vi "test_fpga_ort_fit.vi"() -> ()   [LabVIEW 2016]
uses:
  <vilib>/Platform/TimedLoop/XDataNode/timing_clust.ctl
  <vilib>/Platform/TimedLoop/XDataNode/nitl_modes.ctl
  <vilib>/Platform/TimedLoop/XDataNode/wakeup.ctl
  <vilib>/rvi/Emulation/niFpgaSctlEmulationGetInTimedLoop.vi
  <vilib>/rvi/Emulation/niFpgaEmulationReportErrorSimple.vi
  <vilib>/rvi/Emulation/niFpgaGetClockAttributes.vi
  <vilib>/rvi/Emulation/niFpgaCriticalErrorInLSC.vi
  <vilib>/rvi/Emulation/niFpgaProcessEmulError.vi
  <vilib>/rvi/Emulation/niFpgaEmulationIsFPGAContextNoSignature.vi
  <vilib>/rvi/DataTransferAndStorage/Container/Common/niFpgaContainerGetUniqueNameForEmu.vi
  <vilib>/rvi/Memory/Memory_Emulation/niFpgaMemoryEmulationCacheClearOnFirstRun.vi
  <vilib>/rvi/Memory/Memory_Emulation/nirvimemoryEmulationManagerCache_MakeExclusive.vi
  <vilib>/rvi/Memory/Memory_Emulation/niFpgaMemoryEmulationValidateCache.vi
  <vilib>/rvi/Memory/Memory_Emulation/nirvimemoryEmulationManagerCache_InsertValue.vi
  <vilib>/Utility/error.llb/Clear Errors.vi
  <vilib>/rvi/Memory/Memory_Emulation/nirvimemoryEmulationManagerCache_ReleaseExclusive.vi
  <vilib>/rvi/Memory/Memory_Emulation/nirvimemoryEmulationManagerCache_GetValue.vi
  <vilib>/rvi/Memory/Memory_Emulation/nirvimemoryEmulationManagerCache_SetValue.vi
  <vilib>/rvi/Memory/Memory_Emulation/nirvimemoryFastEmulation.vi
  <vilib>/rvi/Memory/Memory_Emulation/nirvimemoryEmulation.vi
  <vilib>/rvi/errors/nirviReportUnexpectedCaseInternalError (U32).vi
  <vilib>/Platform/TimedLoop/XDataNode/XDataNode.xnode
  <vilib>/rvi/DataTransferAndStorage/Container/XNode/niFpgaContainer.xnode
  <vilib>/rvi/DataTransferAndStorage/Register/Emulation/niFpgaRegisterEmulation.vi
  <vilib>/Platform/TimedLoop/XDataNode/XDNodeRunTimeDep.lvlib
  <vilib>/rvi/FIFO/Fifo_Resource/nirvififoEmulationRead.vi
  <vilib>/rvi/DataTransferAndStorage/Handshake/Emulation/niFpgaHandshakeEmulation.vi
  <vilib>/rvi/FIFO/Fifo_Resource/nirvififoEmulationWrite.vi
panel:
  out "expMABundle":T1
  out "debugOutFitIntermediate":T2
  in  "ort.fit.m.coefficients":T3
  in  "ort.fit.m.weights":T4
  out "paramExtractDebug":cluster{"index":u16, "minimum":i16}
  in  "auxIn":i16
  in  "auxInValid":bool
  in  "inElementValid":bool=TRUE
  in  "inElement":cluster{"index":u16, "data":i16}
  out "debugOutSlopeDissi":T5
  in  "endOfCycle":bool=TRUE
  out "procVar":T6
  in  "ort.fit.p.params":T7={"maxLoc"=0, "threshold"=0, "fitHardPtLimit"=5000}
  in  "ort.p.waveSize":u16=5000
  in  "ort.bgc.p.bgCntP2":u16=12
  out "ort.o.maxIndex":u16
  out "aio.s.ortSubstDeflection":cluster{"index":u16, "data":i16}
  out "ort.o.interactionMax":fxp<+/-,24,16>
  in  "ort.p.fcAvgEnable":bool
  in  "ort.p.fcAvg":i8=-4
  in  "ort.p.methodParams":T8={"ort.p.winSizeP2"=2, "ort.p.syncPoint"=0, "ort.p.useSyncPoint"=FALSE, "ort.p.bypassAvg"=FALSE, "ort.p.searchBounds"={"maxSearchLower"=200, "maxSearchUpper"=600}}
  in  "fb.i.source":u8(ring) items=["Contact Mode", "ORT", "Aux"]
  in  "aio.i.samplingDecimation":u16=1
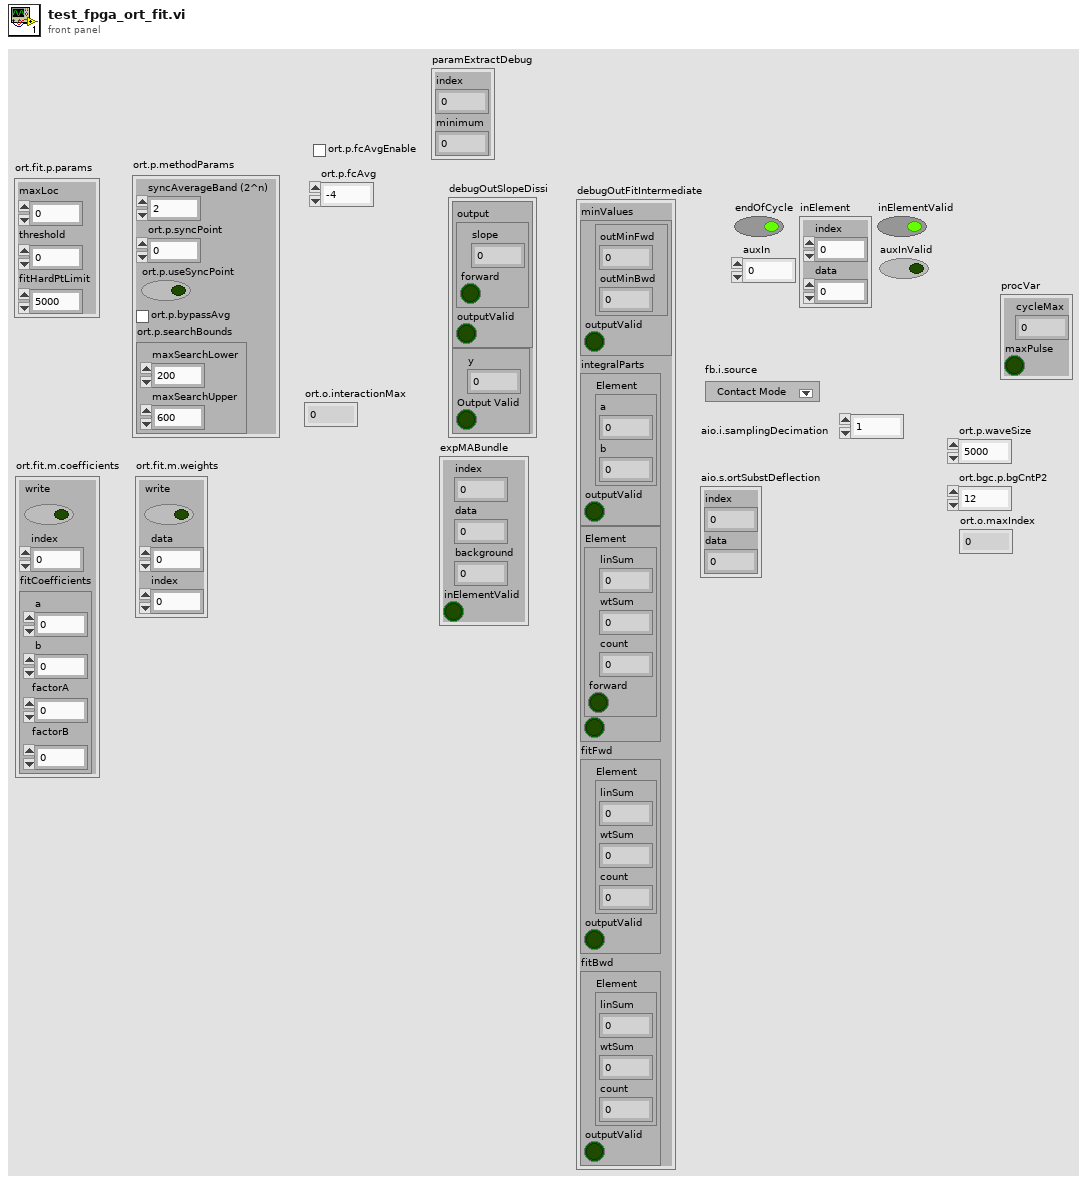
[diagram p1: front panel]
types:
  T1 = cluster{"index":u16, "data":i16, "background":i16, "inElementValid":bool}
  T2 = cluster{"minValues":cluster{cluster{"outMinFwd":fxp<+/-,22,1>, "outMinBwd":fxp<+/-,22,1>}, "outputValid":bool}, "integralParts":cluster{"Element":cluster{"a":i32, "b":i32}, "outputValid":bool}, cluster{"Element":cluster{"linSum":i32, "wtSum":fxp<+/-,54,34>, "count":u16, "forward":bool}, bool}, "fitFwd":cluster{"Element":cluster{"linSum":i32, "wtSum":fxp<+/-,54,34>, "count":u16}, "outputValid":bool}, "fitBwd":cluster{"Element":cluster{"linSum":i32, "wtSum":fxp<+/-,54,34>, "count":u16}, "outputValid":bool}}
  T3 = cluster{"write":bool, "index":u16, "fitCoefficients":cluster{"a":fxp<+/-,21,7>, "b":fxp<+/-,21,7>, "factorA":i8, "factorB":i8}}
  T4 = cluster{"write":bool, "data":fxp<+,20,0>, "index":u16}
  T5 = cluster{cluster{"output":cluster{"slope":fxp<+/-,22,1>, "forward":bool}, "outputValid":bool}, cluster{"y":fxp<+/-,32,1>, "Output Valid":bool}}
  T6 = cluster{"cycleMax":fxp<+/-,24,16>, "maxPulse":bool}
  T7 = cluster{"maxLoc":u16, "threshold":i16, "fitHardPtLimit":u16}
  T8 = cluster{"ort.p.winSizeP2":u16, "ort.p.syncPoint":u16, "ort.p.useSyncPoint":bool, "ort.p.bypassAvg":bool, "ort.p.searchBounds":cluster{"maxSearchLower":u16, "maxSearchUpper":u16}}
  T9 = typedef "XDNodeRunTimeDep.lvlib/timing_clust.ctl" = cluster{"Expected End [f-1]":u64, "Actual End [f-1]":u64, "Finished Late? [f-1]":bool, "Expected End [i-1]":u64, "Actual End [i-1]":u64, "Finished Late? [i-1]":bool, "Expected Start [i]":u64, "Actual Start [i]":u64, "Expected Start [f]":u64, "Actual Start [f]":u64, "Source Name":string, "Structure Name":string, "Period":i64, "Deadline":i64, "Offset":i64, "Start":i64, "Priority":i32, "Timeout":i32, "Mode":T10, "Wakeup Reason":T11, "Error":errorcluster, "Source Type":string, "Secondary Source Type":string, "Global End Time":u64, "Global Start Time":u64, "Frame Duration":u64, "Iteration Duration":u64, "Assigned CPU":i32, "I/O Scan Engine Mode":u32}
  T10 = typedef "XDNodeRunTimeDep.lvlib/nitl_modes.ctl" = enum32{"No Change", "Process missed periods, maintain original phase", "Discard missed periods, maintain original phase", "Process missed periods, ignore original phase", "Discard missed periods, ignore original phase"}
  T11 = typedef "XDNodeRunTimeDep.lvlib/wakeup.ctl" = enum32{"Normal", "Aborted", "Asynchronous wakeup", "Timing source error", "Timed loop error", "Timeout"}
  T12 = cluster{"cycleMax":fxp<+/-,24,16>, "outputValid":bool}
  T13 = cluster{"cycleMax":fxp<+/-,24,16>, "maxPulse":bool}[]
  T14 = cluster{"index":u16, cluster{"data":i16, "background":i16}}
  T15 = cluster{"a":fxp<+/-,21,7>, "b":fxp<+/-,21,7>, "factorA":i8, "factorB":i8}
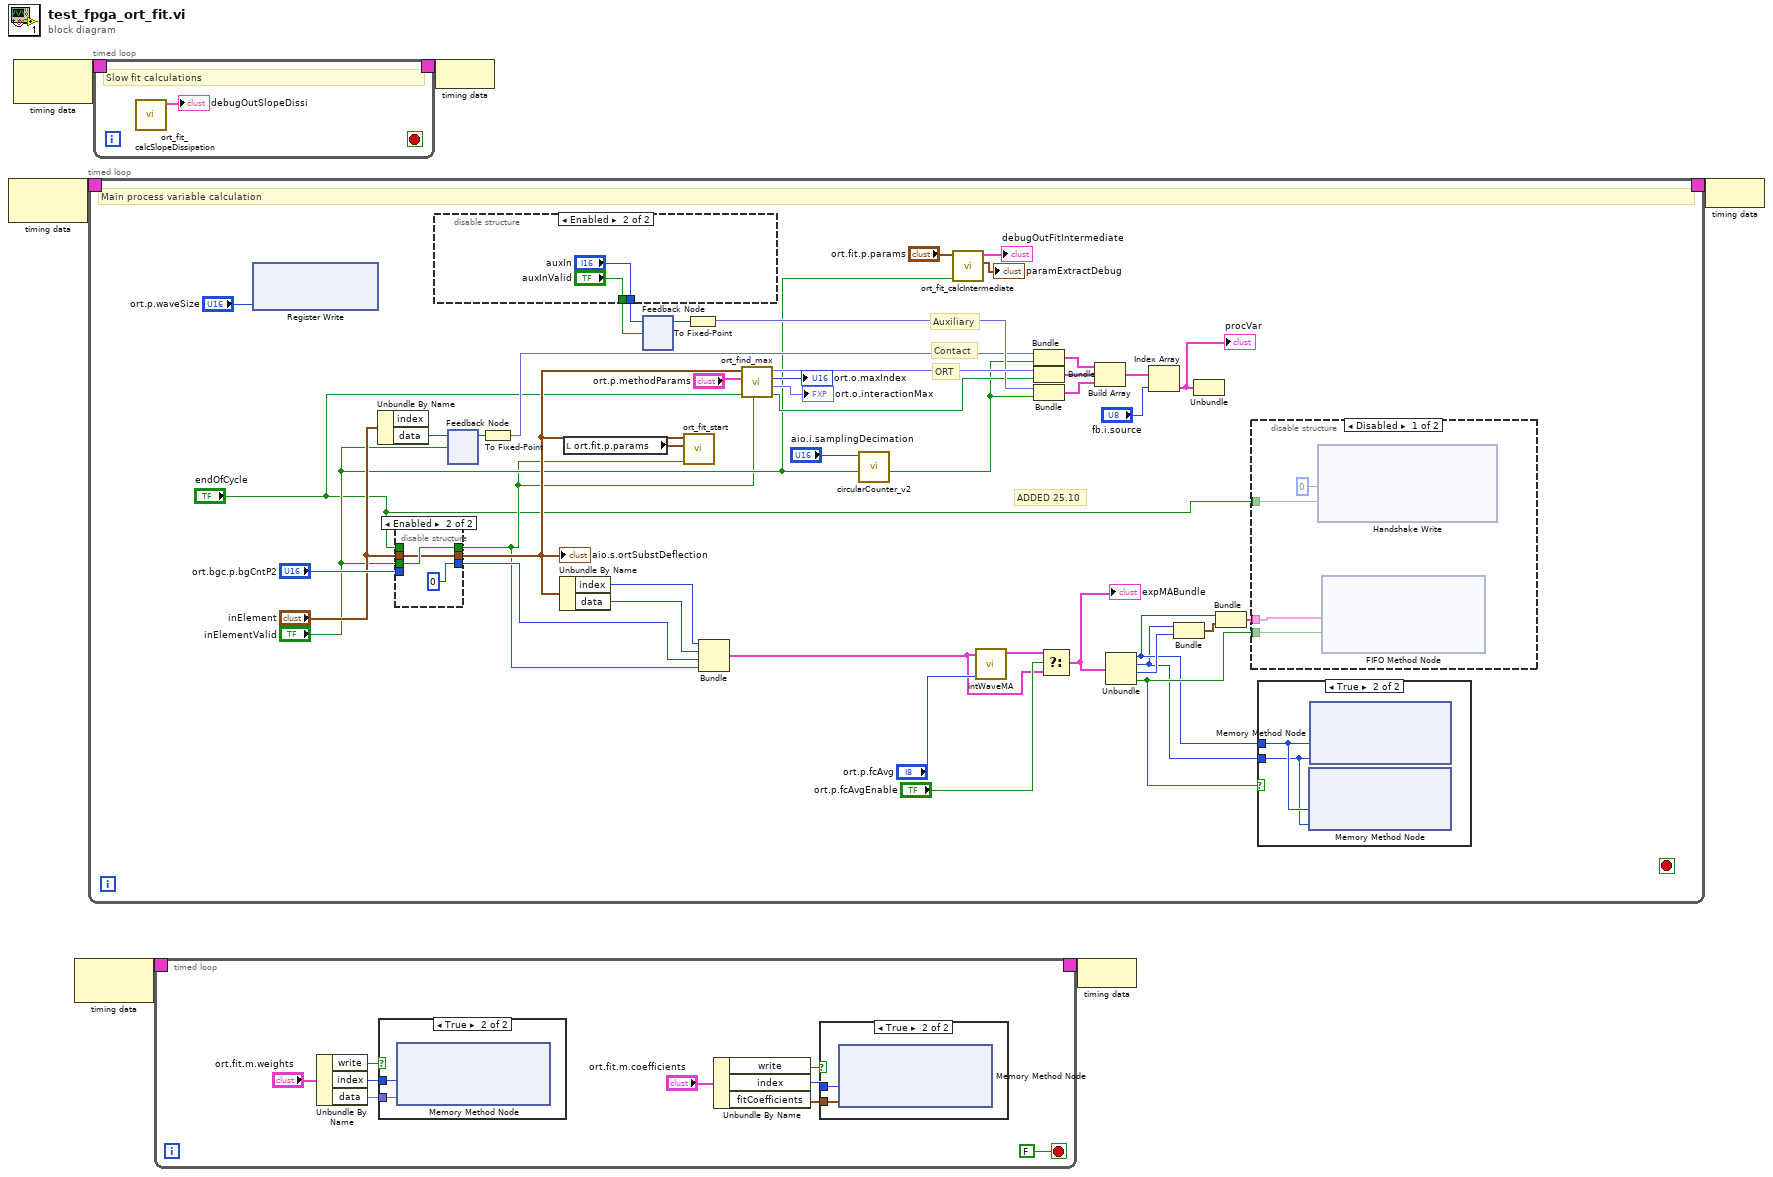
[diagram p0: block diagram]
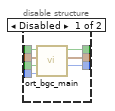
[diagram p4: hidden frame]
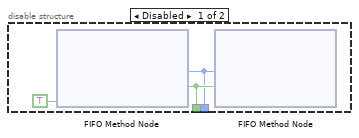
[diagram p5: hidden frame]
diagram:
  n1 = node-c288() -> (w6:T9)  [unwired: 1 in]
  n2 = node-c288() -> (w4:T9)  [unwired: 1 in]
  n3 = node-c288() -> (w2:T9)  [unwired: 1 in]
  n4 = timed-loop {
    timing: w6 -> [_]
    timing-out: [_] -> w5
    stop <- _ stop-if-true
    # "ADDED 25.10"
    # "Auxiliary"
    # "Contact"
    # "ORT"
    # "Main process variable calculation"
    n5 = xnode ("Register Write")("Data"="ort.p.waveSize") -> ()  [unwired: 1 in, 1 out]
    n6 = Unbundle By Name("inElement") -> ("data"=w34:i16)  [unwired: 1 out]
    n7 = disable-structure shown="Enabled" {
      disable-tunnel: [w58 w60] -> w51
      disable-tunnel: [w57 i16 0 ("background")] -> w15
      disable-tunnel: "ort.bgc.p.bgCntP2" -> [w56 _]
      disable-tunnel: [w55 w61] -> w14
      disable-tunnel: "endOfCycle" -> [w54 _]
      disable-tunnel: "inElementValid" -> [w53 w61]
      disable-tunnel: "inElement" -> [w52 w60]
      frame Disabled {
        n8 = call "ort_bgc_main.vi"("ort.bgc.p.bgCntP2"=w56, "inputValid"=w53, "Data"=w52, "endOfWave"=w54) -> ("background"=w57:i16, "output"=w58:cluster{"index":u16, "data":i16}, "outptValid"=w55:bool)  [unwired: 5 in]
      }
      frame Enabled {
      }
    }
    "aio.s.ortSubstDeflection" <- w51
    n9 = disable-structure shown="Enabled" {
      disable-tunnel: [w63 "auxInValid"] -> w50
      disable-tunnel: [w62 "auxIn"] -> w49
      frame Disabled {
        n10 = xnode ("FIFO Method Node")("Ready for Output"=TRUE) -> ("Element"=w62:i16, "Output Valid"=w63:bool)  [unwired: 1 in, 1 out]
        n11 = xnode ("FIFO Method Node")("Element"=w62, "Input Valid"=w63) -> ()  [unwired: 1 in, 2 out]
      }
      frame Enabled {
      }
    }
    n12 = feedback #1() -> (w33:i16)  [unwired: 1 in]
    n13 = feedback-in #1(w34, "inElementValid") -> ()
    n14 = To Fixed-Point(number=w33) -> (fixed-point=w31:fxp<+/-,24,16>)  [unwired: 1 in]
    n15 = Unbundle By Name(w51) -> ("index"=w17:u16, "data"=w16:i16)
    n16 = local read "ort.fit.p.params"() -> (w45:T7)
    n17 = feedback #2() -> (w48:i16)  [unwired: 1 in]
    n18 = feedback-in #2(w49, w50) -> ()
    n19 = call "ort_fit_start.vi"("inputValid"=w14, "ort.fit.p.params"=w45, "data"=w51) -> ()  [unwired: 9 in]
    n20 = To Fixed-Point(number=w48) -> (fixed-point=w40:fxp<+/-,24,16>)  [unwired: 1 in]
    n21 = Bundle("index"=w17, "data"=w16, "background"=w15, "inElementValid"=w14) -> (w13:T1)  [unwired: 1 in]
    n22 = call "ort_find_max.vi"("inputValid"=w14, "endOfCycle"="endOfCycle", "ort.p.methodParams"="ort.p.methodParams", "data"=w51) -> ("outputValid"=w32:bool, "cycleMaxMonitor"=→"ort.o.interactionMax":fxp<+/-,24,16>, "maxIndex"=→"ort.o.maxIndex":u16, "cycleMax"=w41:fxp<+/-,24,16>)  [unwired: 4 in]
    n23 = call "circularCounter_v2.vi"("doStep"="inElementValid", "maxCount"="aio.i.samplingDecimation") -> ("maxPulse"=w28:bool)  [unwired: 6 in, 3 out]
    n24 = call "ort_fit_calcIntermediate.vi"("inputValid"="inElementValid", "ort.fit.p.params"="ort.fit.p.params") -> ("paramExtractDebug"=→"paramExtractDebug":cluster{"index":u16, "minimum":i16}, "output cluster"=→"debugOutFitIntermediate":T2)  [unwired: 8 in]
    n25 = call "intWaveMA.vi"("expFactor"="ort.p.fcAvg", "ortInput"=w13) -> ("ortOutput"=w21:T1)  [unwired: 8 in, 1 out]
    n26 = Bundle(w31, "maxPulse"=w28) -> (w30:cluster{fxp<+/-,24,16>, "maxPulse":bool})  [unwired: 1 in]
    n27 = Bundle("cycleMax"=w41, "outputValid"=w32) -> (w38:T12)  [unwired: 1 in]
    n28 = Bundle(w40, "maxPulse"=w28) -> (w39:cluster{fxp<+/-,24,16>, "maxPulse":bool})  [unwired: 1 in]
    n29 = Select(t=w21, s="ort.p.fcAvgEnable", f=w13) -> (s? t:f=w12:T1)
    "expMABundle" <- w12
    n30 = Build Array(w30, w38, w39) -> (w37:T13)
    n31 = Unbundle(w12) -> ("index"=w8:u16, "data"=w7:i16, "background"=w11:i16, "inElementValid"=w9:bool)
    n32 = Index Array(array=w37, index="fb.i.source") -> (element=w35:T6)
    "procVar" <- w35
    n33 = Bundle("data"=w7, "background"=w11) -> (w22:cluster{"data":i16, "background":i16})  [unwired: 1 in]
    n34 = Unbundle(w35) -> ()  [unwired: 2 out]
    n35 = Bundle("index"=w8, w22) -> (w18:T14)  [unwired: 1 in]
    n36 = disable-structure shown="Disabled" {
      disable-tunnel: "endOfCycle" -> [w70 _]
      disable-tunnel: w18 -> [w68 _]
      disable-tunnel: w9 -> [w67 _]
      frame Disabled {
        n37 = xnode ("Handshake Write")("Data"=u16 0, "Input Valid"=w70) -> ()  [unwired: 1 in, 2 out]
        n38 = xnode ("FIFO Method Node")("Element"=w68, "Input Valid"=w67) -> ()  [unwired: 1 in, 2 out]
      }
      frame Enabled {
      }
    }
    n39 = case shown="True" w9 {
      tunnel: w8 -> [_ w72]
      tunnel: w7 -> [_ w71]
      frame False {
      }
      frame True {
        n40 = xnode ("Memory Method Node")("Address"=w72, "Data"=w71) -> ()  [unwired: 1 in, 1 out]
        n41 = xnode ("Memory Method Node")("Address"=w72, "Data"=w71) -> ()  [unwired: 1 in, 1 out]
      }
    }
  }
  n42 = timed-loop {
    timing: w4 -> [_]
    timing-out: [_] -> w3
    stop <- _ stop-if-true
    # "Slow fit calculations"
    n43 = call "ort_fit_calcSlopeDissipation.vi"() -> ("debugOut"=→"debugOutSlopeDissi":T5)  [unwired: 11 in]
  }
  n44 = timed-loop {
    timing: w2 -> [_]
    timing-out: [_] -> w1
    stop <- FALSE stop-if-true
    n45 = Unbundle By Name("ort.fit.m.weights") -> ("write"=w84:bool, "index"=w85:u16, "data"=w86:fxp<+,20,0>)
    n46 = case shown="True" w84 {
      tunnel: w85 -> [_ w90]
      tunnel: w86 -> [_ w89]
      frame False {
      }
      frame True {
        n47 = xnode ("Memory Method Node")("Address"=w90, "Data"=w89) -> ()  [unwired: 1 in, 1 out]
      }
    }
    n48 = Unbundle By Name("ort.fit.m.coefficients") -> ("write"=w82:bool, "index"=w81:u16, "fitCoefficients"=w79:T15)
    n49 = case shown="True" w82 {
      tunnel: w81 -> [_ w88]
      tunnel: w79 -> [_ w87]
      frame False {
      }
      frame True {
        n50 = xnode ("Memory Method Node")("Address"=w88, "Data"=w87) -> ()  [unwired: 1 in, 1 out]
      }
    }
  }
  n51 = node-c288(w3) -> ()
  n52 = node-c288(w1) -> ()
  n53 = node-c288(w5) -> ()
